vi "standby.vi"(8 "error in (no error)":errorcluster, 11 "MSCU":refnum<class "MSCU.lvclass">) -> (0 "error out":errorcluster, 2 "?":string, 3 "MSCU":refnum<class "MSCU.lvclass">)   [LabVIEW 2019, in "MSCU.lvclass"]
uses:
  MSCU.lvclass
  MSCU.lvclass/MSCU.ctl
panel:
  in  "Mode":i32 min=-1 max=0 step=1
  # "1 = enter standby\n0 = exit standby"
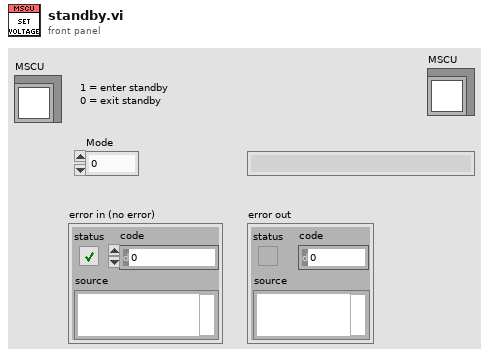
[diagram p1: front panel]
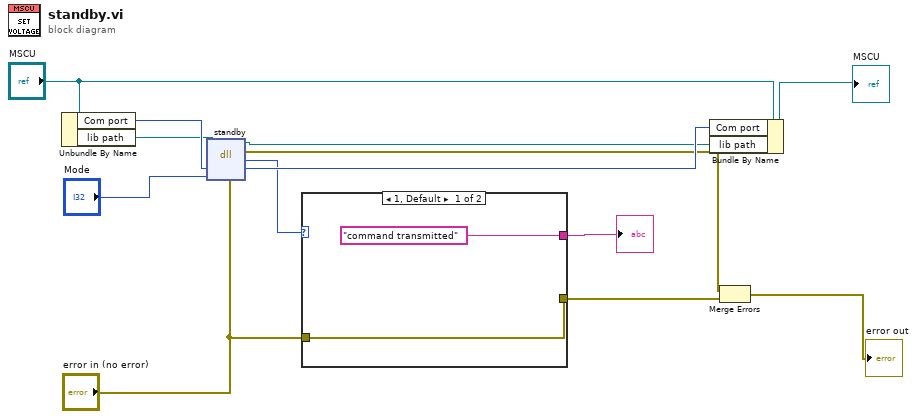
[diagram p0: block diagram]
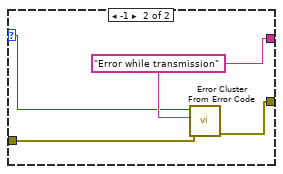
[diagram p2: hidden frame]
diagram:
  n1 = Unbundle By Name("MSCU") -> ("Com port"=w10:i32, "lib path"=w9:path)
  n2 = dll-call lib="C:/Program Files (x86)/Nanonis/SPM Controller/data/MSCU.dll" fn="standby"(path in=w9, error in="error in (no error)", "Comport"=w10, "Mode"="Mode") -> (path out=w7:path, error out=w5:errorcluster, "return type"=w11:i32, "Comport"=w13:i32)  [unwired: 2 in]
  n3 = case shown="1, Default" w11 {
    selector: w11 -> [_ w16]
    tunnel: ["command transmitted" w17] -> w12
    tunnel: [w14 w18] -> w3
    tunnel: "error in (no error)" -> [w14 w19]
    frame 1, Default {
    }
    frame -1 {
      w17 = "Error while transmission"
      n4 = call <vilib>:"Error Cluster From Error Code.vi"("error in (no error)"=w19, "error message (\"\")"=w17, "error code (0)"=w16) -> ("error out"=w18:errorcluster)  [unwired: 6 in]
    }
  }
  "?" <- w12
  n5 = Bundle By Name(cluster="MSCU", "Com port"=w13, "lib path"=w7) -> (→"MSCU":refnum<class "MSCU.lvclass">)
  n6 = Merge Errors(w5, w3) -> (→"error out":errorcluster)
